vi "Circular Buffer(2D I16).vi"(7 "Buffer Size":T3, 8 "error in (no error)":errorcluster, 9 "Read Size":i32, 10 "Operation":T1, 11 "Data In":i16[][](array[numeric])) -> (0 "error out":errorcluster, 1 "Elements Remaining":i32, 2 "Buffer Status":T2, 3 "Data Out":i16[][](array[numeric]))   [LabVIEW 2020, in "Circular Buffer.lvlib"]
doc: "This VI implements a circular buffer which data can be written to and read from. There can only be one buffer per data type at once, but you can have multiple buffers of different types at the same time. For example, you can have a buffer of Wfm data types as well as I32s in the same VI. You cannot have two independent buffers of I32s."
uses:
  Circular Buffer.lvlib
  Controls/Circular Buffer Status.ctl
  Controls/Circular Buffer Operations.ctl
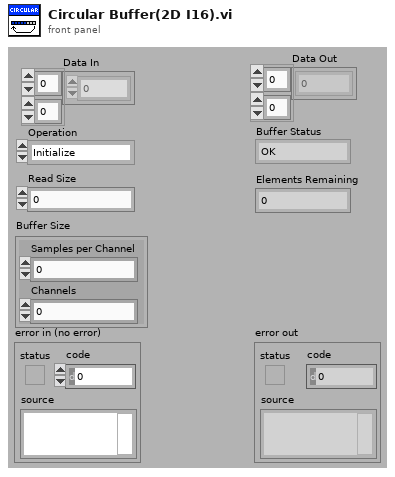
[diagram p1: front panel]
types:
  T1 = typedef "Circular Buffer.lvlib/Circular Buffer Operations.ctl" = enum16{"Initialize", "Get Backlog", "Write", "Read (continuous)", "Read (most recent)"}
  T2 = typedef "Circular Buffer.lvlib/Circular Buffer Status.ctl" = enum16{"OK", "Overflow", "Underflow"}
  T3 = cluster{"Samples per Channel":u32, "Channels":u32}
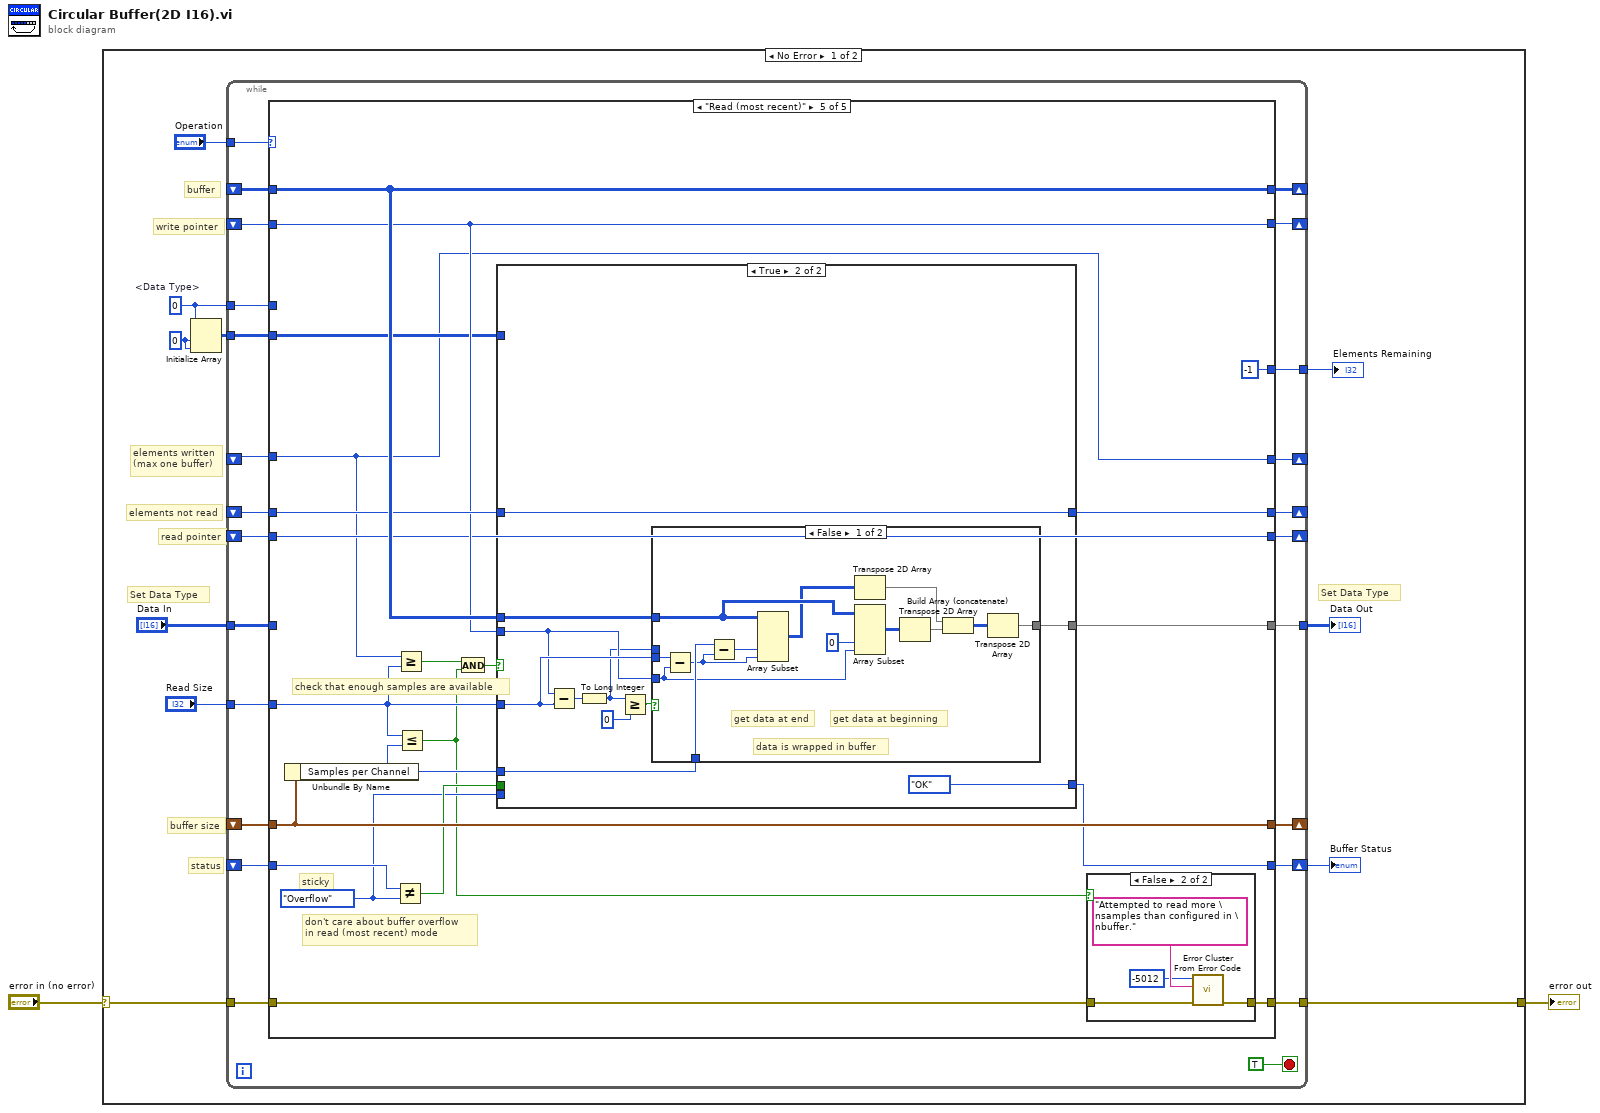
[diagram p0: block diagram]
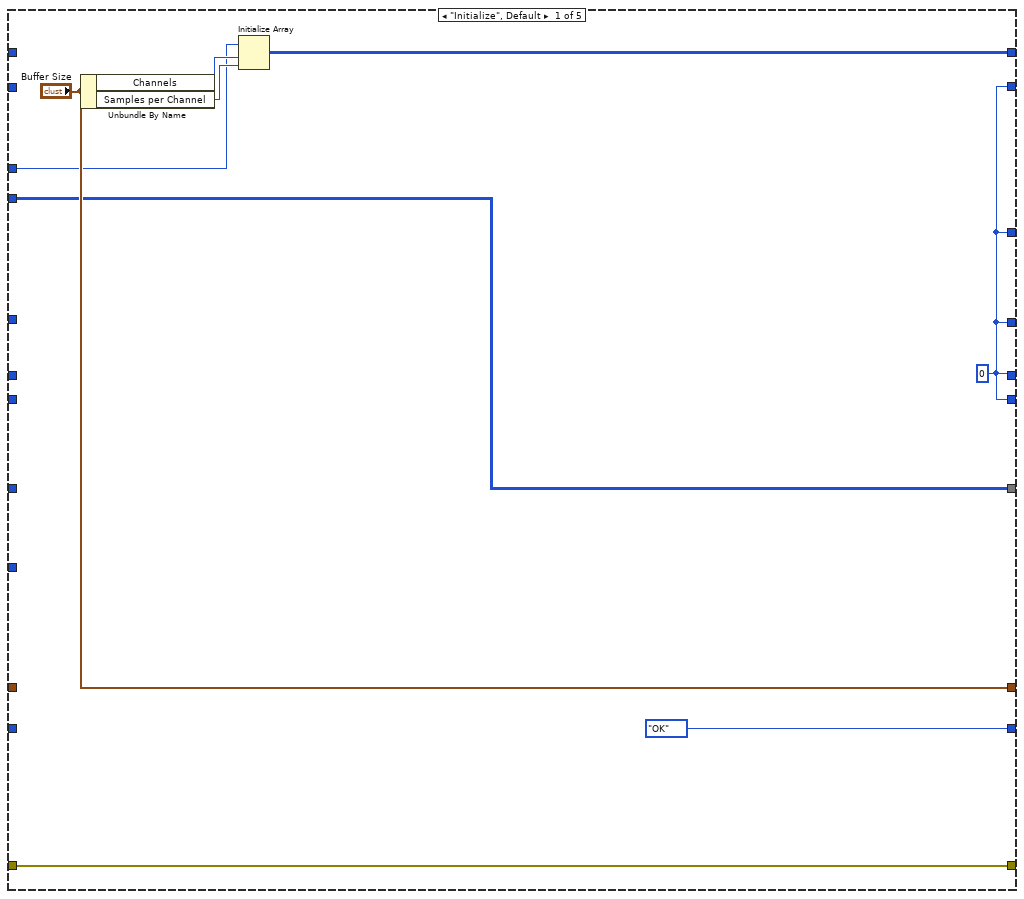
[diagram p2: hidden frame]
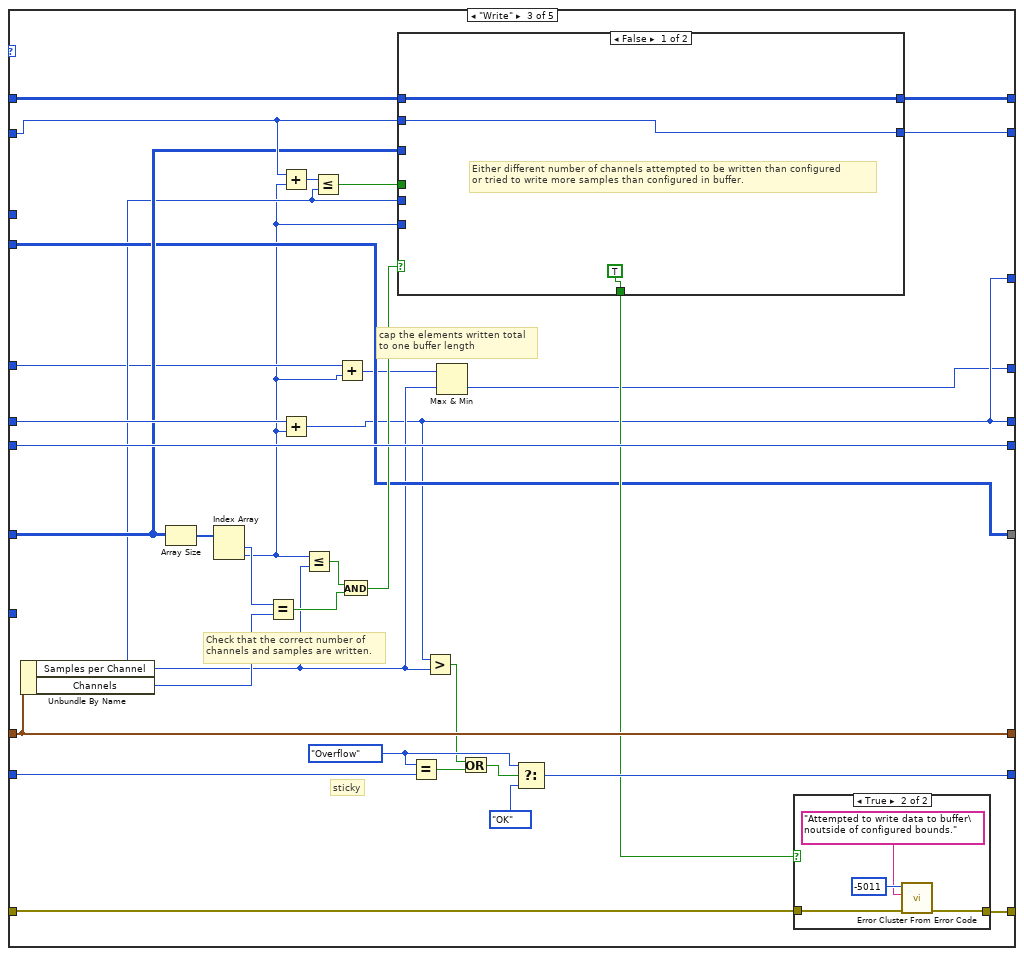
[diagram p4: hidden frame]
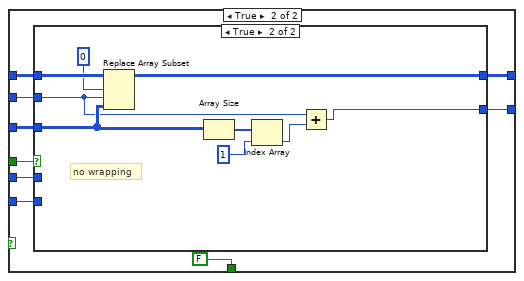
[diagram p6: hidden frame]
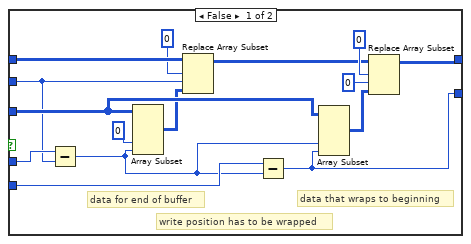
[diagram p7: hidden frame]
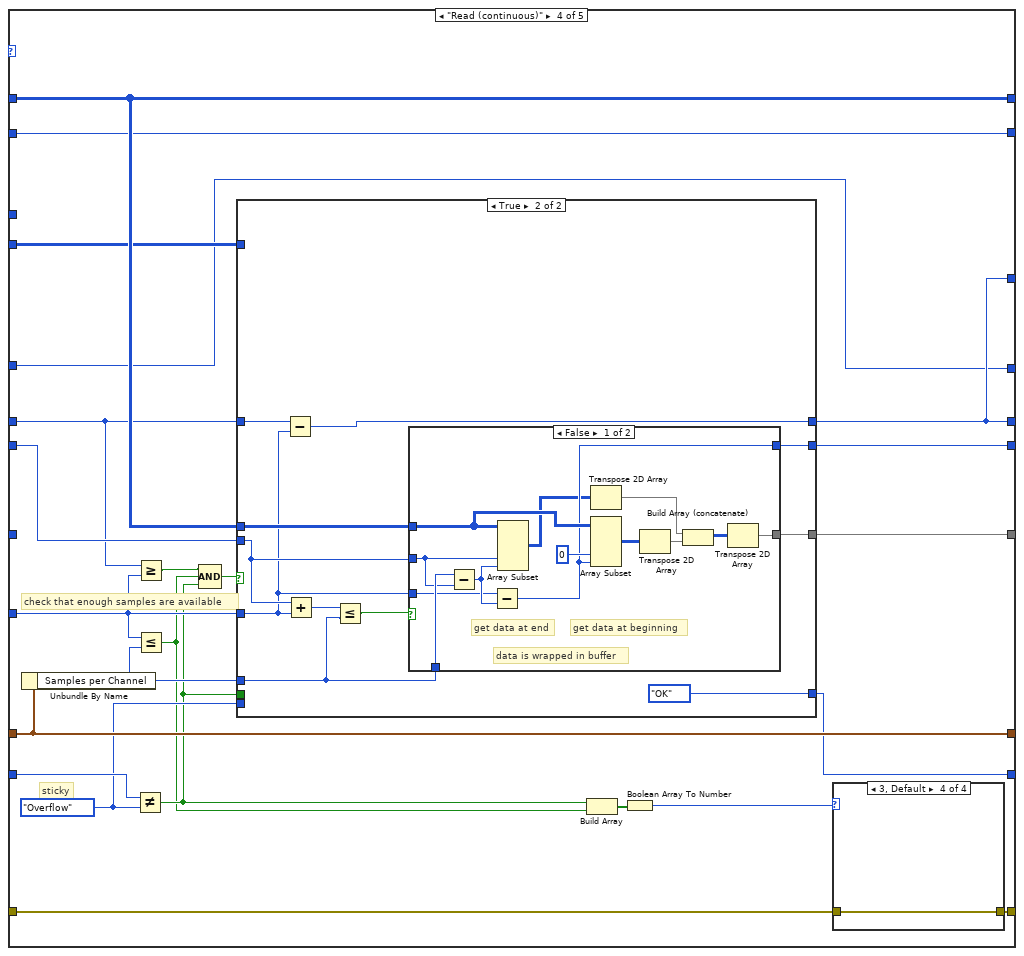
[diagram p8: hidden frame]
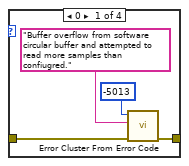
[diagram p9: hidden frame]
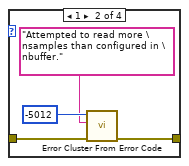
[diagram p10: hidden frame]
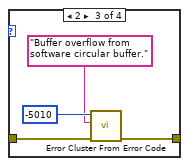
[diagram p11: hidden frame]
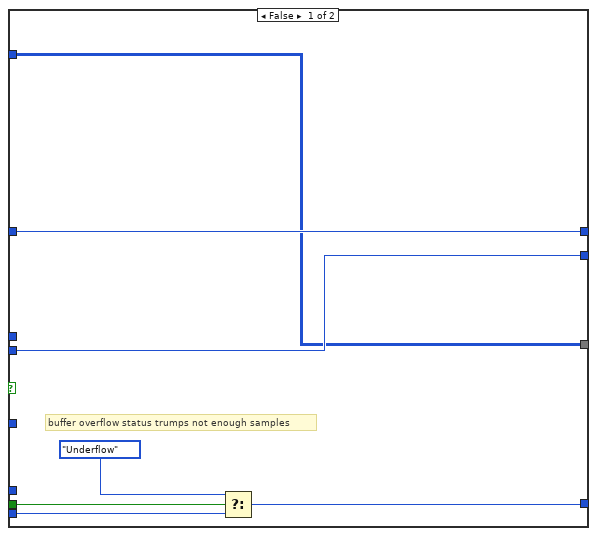
[diagram p12: hidden frame]
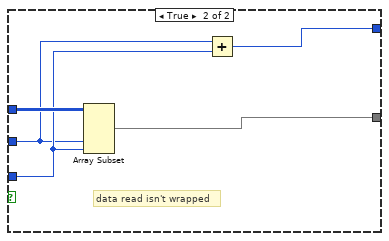
[diagram p13: hidden frame]
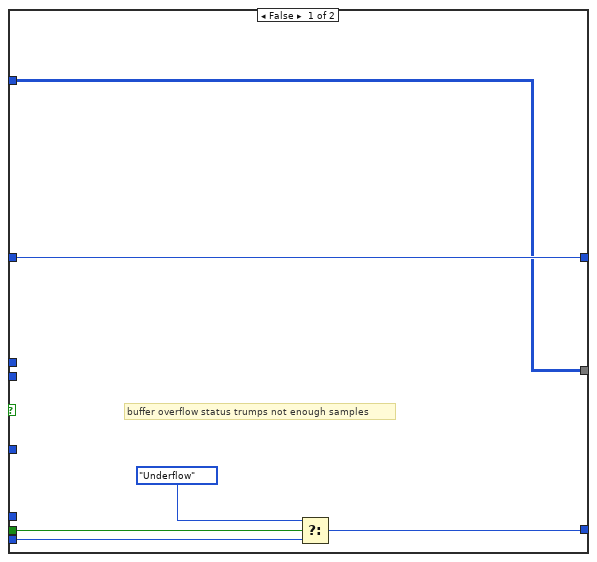
[diagram p15: hidden frame]
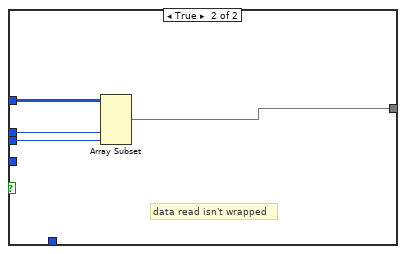
[diagram p16: hidden frame]
diagram:
  n1 = case shown="No Error" "error in (no error)" {
    selector: "error in (no error)" -> [w8 w262]
    tunnel: [w7 w262] -> w1
    frame No Error {
      w6 = i16 0  # <Data Type>
      w5 = 0 ("dimension size")
      # "elements written\n(max one buffer)"
      # "Set Data Type"
      # "Set Data Type"
      # "write pointer"
      # "status"
      # "buffer size"
      # "read pointer"
      # "elements not read"
      # "buffer"
      n2 = Initialize Array(w6, w5, w5) -> (w4:i16[][])
      n3 = while {
        tunnel: "Operation" -> [w36]
        shift-right: [w35] -> _
        shift-left: _ -> [w32]
        shift-right: [w34] -> _
        shift-left: _ -> [w30]
        shift-right: [w33] -> _
        shift-left: _ -> [w27]
        tunnel: "Data In" -> [w31]
        shift-right: [w29] -> _
        shift-left: _ -> [w28]
        tunnel: "Read Size" -> [w26]
        shift-right: [w25] -> w10
        shift-left: _ -> [w24]
        tunnel: [w23] -> w11
        tunnel: [w22] -> w7
        tunnel: w8 -> [w21]
        shift-right: [w20] -> _
        shift-left: _ -> [w19]
        tunnel: w6 -> [w18]
        tunnel: w4 -> [w17]
        tunnel: [w16] -> w3
        shift-right: [w14] -> _
        shift-left: _ -> [w15]
        stop <- TRUE stop-if-true
        n4 = case shown="\"Read (most recent)\"" w36 {
          tunnel: [w46 w54 w65 w152 w222] -> w35
          tunnel: [w38 w48 w58 w131 w217] -> w34
          tunnel: [w38 w52 w82 w148 w212] -> w33
          tunnel: w32 -> [_ w54 w64 w152 w222]
          tunnel: w31 -> [_ _ w74 _ _]
          tunnel: w30 -> [_ w48 w79 w132 w215]
          tunnel: ["Buffer Size" w53 w88 w151 w221] -> w29
          tunnel: w28 -> [_ w53 w88 w151 w221]
          tunnel: w27 -> [_ w52 w82 w147 w212]
          tunnel: w26 -> [_ _ _ w141 w209]
          tunnel: [Circular_Buffer_Status."OK" ("status") w50 w87 w146 w216] -> w25
          tunnel: w24 -> [_ w50 w84 w150 w220]
          tunnel: [w39 w49 w63 w142 w214] -> w23
          tunnel: [w41 w55 w72 w145 w210] -> w22
          tunnel: w21 -> [w41 w55 w71 w144 w211]
          tunnel: [w38 w51 w76 w143 w213] -> w20
          tunnel: w19 -> [_ w51 w75 w143 w213]
          tunnel: w18 -> [w40 _ _ _ _]
          tunnel: w17 -> [w39 w49 w63 w133 w204]
          tunnel: [w38 w48 w58 w131 -1] -> w16
          tunnel: w15 -> [_ w47 w59 w130 w202]
          tunnel: [w38 w47 w56 w130 w202] -> w14
          frame "Initialize", Default {
            w38 = 0 ("dimension size 2")
            n5 = Unbundle By Name("Buffer Size") -> ("Channels"=w43:u32, "Samples per Channel"=w42:u32)
            n6 = Initialize Array(w40, w43, w42) -> (w46:i16[][])
          }
          frame "Get Backlog" {
          }
          frame "Write" {
            w83 = Circular_Buffer_Status."Overflow" ("status")
            # "cap the elements written total\nto one buffer length"
            # "Check that the correct number of\nchannels and samples are written."
            # "sticky"
            n7 = Unbundle By Name(w88) -> ("Samples per Channel"=w60:u32, "Channels"=w69:u32)
            n8 = Array Size(array=w74) -> (size(s)=w73:i32[])
            n9 = Index Array(array=w73) -> (element #1=w62:i32, element #2=w57:i32)  [unwired: 2 in]
            n10 = Equal?(x=w62, y=w69) -> (x = y?=w67:bool)
            n11 = Add(x=w75, y=w57) -> (x+y=w78:u32)
            n12 = Add(x=w79, y=w57) -> (x+y=w58:i32)
            n13 = Less Or Equal?(x=w57, y=w60) -> (x <= y?=w68:bool)
            n14 = Less Or Equal?(x=w78, y=w60) -> (x <= y?=w77:bool)
            n15 = Add(x=w59, y=w57) -> (x+y=w61:u32)
            n16 = And(x=w68, y=w67) -> (x .and. y?=w66:bool)
            n17 = case shown="False" w66 {
              tunnel: [w96 w105] -> w65
              tunnel: w77 -> [_ w104]
              tunnel: [w95 w103] -> w76
              tunnel: w75 -> [w95 w102]
              tunnel: w64 -> [w96 w101]
              tunnel: w74 -> [_ w100]
              tunnel: w57 -> [_ w99]
              tunnel: w60 -> [_ w98]
              tunnel: [TRUE FALSE] -> w70
              frame False {
                # "Either different number of channels attempted to be written than configured\nor tried to write more samples than configured in buffer."
              }
              frame True {
                n18 = case shown="True" w104 {
                  tunnel: w101 -> [w120 w129]
                  tunnel: [w115 w127] -> w105
                  tunnel: w102 -> [w109 w122]
                  tunnel: w100 -> [w113 w124]
                  tunnel: w98 -> [w110 _]
                  tunnel: w99 -> [w112 _]
                  tunnel: [w111 w121] -> w103
                  frame False {
                    # "data that wraps to beginning"
                    # "data for end of buffer"
                    # "write position has to be wrapped"
                    n19 = Subtract(x=w110, y=w109) -> (x-y=w108:u32)
                    n20 = Array Subset(array=w113, index (col)=0 ("index"), length (col)=w108) -> (w107:i16[][])  [unwired: 2 in]
                    n21 = Replace Array Subset(array=w120, new element=w107, index (row)=0, index (col)=w109) -> (w116:i16[][])
                    n22 = Subtract(x=w112, y=w108) -> (x-y=w111:u32)
                    n23 = Array Subset(array=w113, index (col)=w108, length (col)=w111) -> (w118:i16[][])  [unwired: 2 in]
                    n24 = Replace Array Subset(array=w116, new element=w118, index (row)=0, index (col)=0 ("disabled index (col)")) -> (w115:i16[][])
                  }
                  frame True {
                    # "no wrapping"
                    n25 = Replace Array Subset(array=w129, new element=w124, index (row)=0 ("disabled index (col)"), index (col)=w122) -> (w127:i16[][])
                    n26 = Array Size(array=w124) -> (size(s)=w126:i32[])
                    n27 = Index Array(array=w126, index=1) -> (element=w123:i32)
                    n28 = Add(x=w122, y=w123) -> (x+y=w121:u32)
                  }
                }
              }
            }
            n29 = Equal?(x=w83, y=w84) -> (x = y?=w86:bool)
            n30 = Greater?(x=w58, y=w60) -> (0:w81:bool)
            n31 = Max & Min(x=w61, y=w60) -> (min(x,y)=w56:u32)  [unwired: 1 out]
            n32 = Or(x=w81, y=w86) -> (x .or. y?=w85:bool)
            n33 = Select(t=w83, s=w85, f=Circular_Buffer_Status."OK" ("status")) -> (s? t:f=w87:T2)
            n34 = case shown="True" w70 {
              tunnel: w71 -> [w89 w92]
              tunnel: [w89 w91] -> w72
              frame False {
              }
              frame True {
                n35 = call <vilib>:"Error Cluster From Error Code.vi"("error in (no error)"=w92, "error message (\"\")"="Attempted to write data to buffer\noutside of configured bounds.", "error code (0)"=-5011 ("code")) -> ("error out"=w91:errorcluster)  [unwired: 1 in, 5 out]
              }
            }
          }
          frame "Read (continuous)" {
            w149 = Circular_Buffer_Status."Overflow" ("status")
            # "check that enough samples are available"
            # "sticky"
            n36 = Unbundle By Name(w151) -> ("Samples per Channel"=w140:u32)
            n37 = Not Equal?(x=w150, y=w149) -> (x != y?=w137:bool)
            n38 = Greater Or Equal?(x=w132, y=w141) -> (x >= y?=w139:bool)
            n39 = Less Or Equal?(x=w141, y=w140) -> (x <= y?=w136:bool)
            n40 = Compound Arithmetic op=AND(w139, w136, w137) -> (w138:bool)
            n41 = case shown="True" w138 {
              tunnel: w147 -> [w167 w176]
              tunnel: w152 -> [_ w182]
              tunnel: w141 -> [_ w175]
              tunnel: w140 -> [_ w177]
              tunnel: [w171 Circular_Buffer_Status."OK" ("status")] -> w146
              tunnel: w137 -> [w172 _]
              tunnel: w149 -> [w170 _]
              tunnel: w132 -> [w168 w174]
              tunnel: [w168 w173] -> w131
              tunnel: [w167 w178] -> w148
              tunnel: [w166 w179] -> w142
              tunnel: w133 -> [w166 _]
              frame False {
                # "buffer overflow status trumps not enough samples"
                n42 = Select(t=Circular_Buffer_Status."Underflow" ("status"), s=w172, f=w170) -> (s? t:f=w171:T2)
              }
              frame True {
                n43 = Subtract(x=w174, y=w175) -> (x-y=w173:i32)
                n44 = Add(x=w176, y=w175) -> (x+y=w181:u32)
                n45 = Less Or Equal?(x=w181, y=w177) -> (x <= y?=w180:bool)
                n46 = case shown="False" w180 {
                  tunnel: w182 -> [w195 w201]
                  tunnel: w176 -> [w191 w198]
                  tunnel: w175 -> [w184 w199]
                  tunnel: [w186 w200] -> w179
                  tunnel: [w192 w197] -> w178
                  tunnel: w177 -> [w196 _]
                  frame False {
                    # "get data at beginning"
                    # "get data at end"
                    # "data is wrapped in buffer"
                    n47 = Subtract(x=w196, y=w191) -> (x-y=w193:u32)
                    n48 = Subtract(x=w184, y=w193) -> (x-y=w192:u32)
                    n49 = Array Subset(array=w195, index (col)=w191, length (col)=w193) -> (w190:i16[][])  [unwired: 2 in]
                    n50 = Transpose 2D Array(2D array=w190) -> (transposed array=w188:i16[][])
                    n51 = Array Subset(array=w195, index (col)=0 ("index"), length (col)=w192) -> (w189:i16[][])  [unwired: 2 in]
                    n52 = Transpose 2D Array(2D array=w189) -> (transposed array=w187:i16[][])
                    n53 = Build Array (concatenate)(w188, w187) -> (w185:i16[][])
                    n54 = Transpose 2D Array(2D array=w185) -> (transposed array=w186:i16[][])
                  }
                  frame True {
                    # "data read isn't wrapped"
                    n55 = Array Subset(array=w201, index (col)=w198, length (col)=w199) -> (w200:i16[][])  [unwired: 2 in]
                    n56 = Add(x=w198, y=w199) -> (x+y=w197:u32)
                  }
                }
              }
            }
            n57 = Build Array(w137, w136) -> (w135:bool[])
            n58 = Boolean Array To Number(Boolean array=w135) -> (number=w134:u32)
            n59 = case shown="3, Default" w134 {
              tunnel: w144 -> [w156 w160 w164 w165]
              tunnel: [w155 w159 w163 w165] -> w145
              frame 0 {
                n60 = call <vilib>:"Error Cluster From Error Code.vi"("error in (no error)"=w156, "error message (\"\")"="Buffer overflow from software circular buffer and attempted to read more samples than confiugred.", "error code (0)"=-5013 ("code")) -> ("error out"=w155:errorcluster)  [unwired: 1 in, 5 out]
              }
              frame 1 {
                n61 = call <vilib>:"Error Cluster From Error Code.vi"("error in (no error)"=w160, "error message (\"\")"="Attempted to read more \nsamples than configured in \nbuffer.", "error code (0)"=-5012 ("code")) -> ("error out"=w159:errorcluster)  [unwired: 2 in, 4 out]
              }
              frame 2 {
                n62 = call <vilib>:"Error Cluster From Error Code.vi"("error in (no error)"=w164, "error message (\"\")"="Buffer overflow from software circular buffer.", "error code (0)"=-5010 ("code")) -> ("error out"=w163:errorcluster)  [unwired: 1 in, 5 out]
              }
              frame 3, Default {
              }
            }
          }
          frame "Read (most recent)" {
            w218 = Circular_Buffer_Status."Overflow" ("status")
            # "don't care about buffer overflow\nin read (most recent) mode"
            # "check that enough samples are available"
            # "sticky"
            n63 = Unbundle By Name(w221) -> ("Samples per Channel"=w208:u32)
            n64 = Not Equal?(x=w220, y=w218) -> (x != y?=w219:bool)
            n65 = Greater Or Equal?(x=w202, y=w209) -> (x >= y?=w206:bool)
            n66 = Less Or Equal?(x=w209, y=w208) -> (x <= y?=w205:bool)
            n67 = And(x=w206, y=w205) -> (x .and. y?=w207:bool)
            n68 = case shown="True" w207 {
              tunnel: w213 -> [_ w236]
              tunnel: w222 -> [_ w242]
              tunnel: w209 -> [_ w238]
              tunnel: w208 -> [_ w239]
              tunnel: [w232 Circular_Buffer_Status."OK" ("status")] -> w216
              tunnel: w219 -> [w233 _]
              tunnel: w218 -> [w231 _]
              tunnel: w215 -> [w229 w243]
              tunnel: [w229 w243] -> w217
              tunnel: [w228 w240] -> w214
              tunnel: w204 -> [w228 _]
              frame False {
                # "buffer overflow status trumps not enough samples"
                n69 = Select(t=Circular_Buffer_Status."Underflow" ("status"), s=w233, f=w231) -> (s? t:f=w232:T2)
              }
              frame True {
                n70 = Subtract(x=w236, y=w238) -> (x-y=w235:u32)
                n71 = To Long Integer(number=w235) -> (32bit integer=w234:i32)
                n72 = Greater Or Equal?(x=w234, y=0) -> (x >= y?=w241:bool)
                n73 = case shown="False" w241 {
                  tunnel: w242 -> [w256 w261]
                  tunnel: [w250 w260] -> w240
                  tunnel: w239 -> [w257 _]
                  tunnel: w234 -> [_ w259]
                  tunnel: w238 -> [w248 w258]
                  tunnel: w236 -> [w245 _]
                  frame False {
                    # "get data at beginning"
                    # "get data at end"
                    # "data is wrapped in buffer"
                    n74 = Subtract(x=w248, y=w245) -> (x-y=w246:u32)
                    n75 = Subtract(x=w257, y=w246) -> (x-y=w247:u32)
                    n76 = Array Subset(array=w256, index (col)=w247, length (col)=w246) -> (w254:i16[][])  [unwired: 2 in]
                    n77 = Transpose 2D Array(2D array=w254) -> (transposed array=w252:i16[][])
                    n78 = Array Subset(array=w256, index (col)=0 ("index"), length (col)=w245) -> (w253:i16[][])  [unwired: 2 in]
                    n79 = Transpose 2D Array(2D array=w253) -> (transposed array=w251:i16[][])
                    n80 = Build Array (concatenate)(w252, w251) -> (w249:i16[][])
                    n81 = Transpose 2D Array(2D array=w249) -> (transposed array=w250:i16[][])
                  }
                  frame True {
                    # "data read isn't wrapped"
                    n82 = Array Subset(array=w261, index (col)=w259, length (col)=w258) -> (w260:i16[][])  [unwired: 2 in]
                  }
                }
              }
            }
            n83 = case shown="False" w205 {
              tunnel: w211 -> [w223 w225]
              tunnel: [w223 w224] -> w210
              frame True {
              }
              frame False {
                n84 = call <vilib>:"Error Cluster From Error Code.vi"("error in (no error)"=w225, "error message (\"\")"="Attempted to read more \nsamples than configured in \nbuffer.", "error code (0)"=-5012 ("code")) -> ("error out"=w224:errorcluster)  [unwired: 1 in, 5 out]
              }
            }
          }
        }
      }
      "Elements Remaining" <- w3
      "Data Out" <- w11
      "Buffer Status" <- w10
    }
    frame Error {
    }
  }
  "error out" <- w1
